vi "Source Distribution Builder.vi"(8 "error in (no error)":errorcluster, 10 "Build Specifications":string[](array[string]), 11 "Path to project":path) -> (0 "error out":errorcluster, 2 "Generated files":path[][](array[path]), 3 "Path to project out":path)   [LabVIEW 2019, in "Package Builder.lvlib"]
uses:
  Package Builder.lvlib
  <vilib>/AppBuilder/AB_API_Simple/Build (path).vi
  <vilib>/AppBuilder/AB_API_Simple/NI_App_Builder_API.lvlib
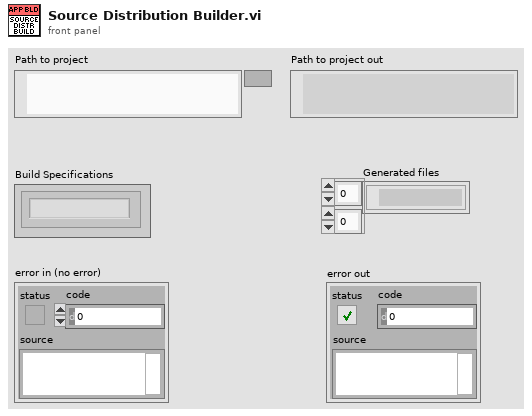
[diagram p1: front panel]
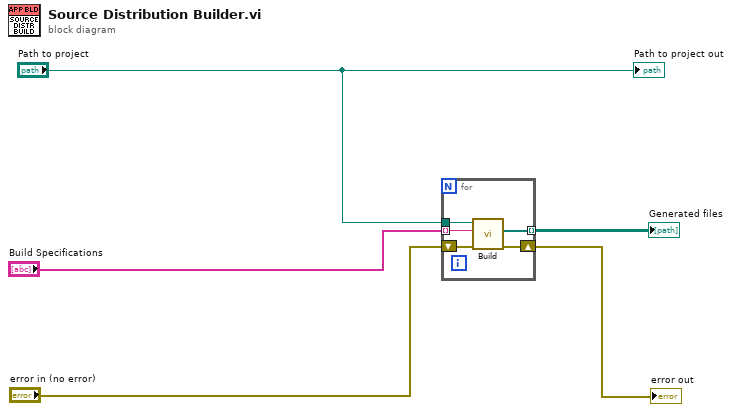
[diagram p0: block diagram]
diagram:
  n1 = for {
    tunnel: "Path to project" -> [w10]
    shift-right: [w8] -> w2
    shift-left: "error in (no error)" -> [w9]
    tunnel: "Build Specifications" -> [w7] mode=indexing
    tunnel: [w6] -> w1 mode=indexing
    n2 = call-poly <vilib>:"Build.vi"("error in (no error)"=w9, "Name of build specification (if empty: build all)"=w7, "Path to project"=w10) -> ("error out"=w8:errorcluster, "Generated files"=w6:path[])  [unwired: 7 in]
  }
  "error out" <- w2
  "Generated files" <- w1
  "Path to project out" <- "Path to project"
